vi "ReadMultipleDigitalOutputs.vi"(8 "error in (no error)":errorcluster, 11 "TesteractHAL_DigitalOutput_NIDAQmx In":refnum<class "TesteractHAL_DigitalOutput_NIDAQmx.lvclass">) -> (0 "error out":errorcluster, 2 "data":bool[](array[boolean]), 3 "TesteractHAL_DigitalOutput_NIDAQmx Out":refnum<class "TesteractHAL_DigitalOutput_NIDAQmx.lvclass">)   [LabVIEW 2017, in "TesteractHAL_DigitalOutput_NIDAQmx.lvlib" / "TesteractHAL_DigitalOutput_NIDAQmx.lvclass"]
doc: "Read multiple lines as booleans"
uses:
  TesteractHAL_DigitalOutput_NIDAQmx.lvclass
  TesteractHAL_DigitalOutput_NIDAQmx.lvclass/TesteractHAL_DigitalOutput_NIDAQmx.ctl
  <vilib>/DAQmx/read.llb/DAQmx Read (Digital Bool 1Line 1Point).vi
  <vilib>/DAQmx/create/channels.llb/DAQmx Create Channel (DO-Digital Output).vi
  <vilib>/DAQmx/miscellaneous.llb/DAQmx Fill In Error Info.vi
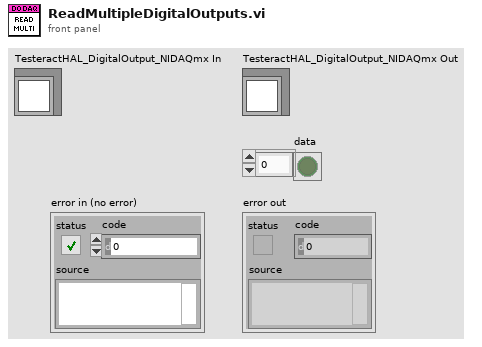
[diagram p1: front panel]
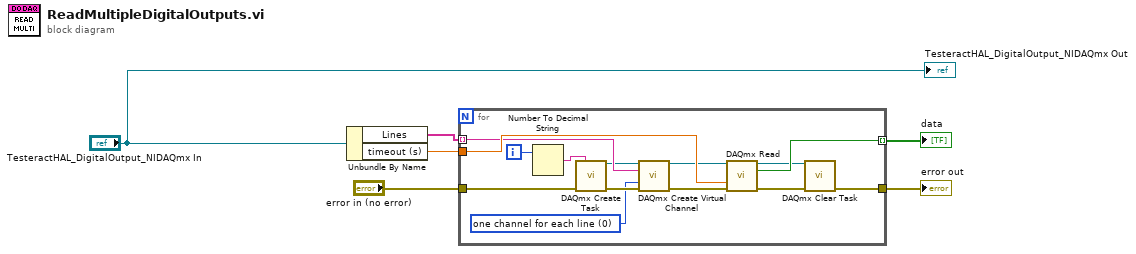
[diagram p0: block diagram]
diagram:
  n1 = Unbundle By Name("TesteractHAL_DigitalOutput_NIDAQmx In") -> ("Lines"=w3:string[], "timeout (s)"=w2:dbl)
  n2 = for {
    tunnel: [w17] -> w6
    tunnel: [w19] -> w5 mode=indexing
    tunnel: w3 -> [w11] mode=indexing
    tunnel: w2 -> [w18]
    tunnel: "error in (no error)" -> [w9]
    i -> [w13]
    w7 = 0 items=["one channel for each line", "one channel for all lines"] ("line grouping")
    n3 = Number To Decimal String(number=w13) -> (decimal integer string=w12:string)  [unwired: 1 in]
    n4 = call <vilib>:"DAQmx Create Task.vi"("new task name"=w12, "error in"=w9) -> ("task out"=w10:refnum<k21>, "error out"=w8:errorcluster)  [unwired: 12 in]
    n5 = call-poly <vilib>:"DAQmx Create Virtual Channel.vi"("task in"=w10, "lines"=w11, "line grouping"=w7, "error in"=w8) -> ("task out"=w14:refnum<k21>, "error out"=w15:errorcluster)  [unwired: 10 in]
    n6 = call-poly <vilib>:"DAQmx Read.vi"("task/channels in"=w14, "timeout"=w18, "error in"=w15) -> ("task out"=w16:refnum<k21>, "data"=w19:bool, "error out"=w20:errorcluster)  [unwired: 10 in]
    n7 = call <vilib>:"DAQmx Clear Task.vi"("task in"=w16, "error in"=w20) -> ("error out"=w17:errorcluster)  [unwired: 13 in]
  }
  "error out" <- w6
  "data" <- w5
  "TesteractHAL_DigitalOutput_NIDAQmx Out" <- "TesteractHAL_DigitalOutput_NIDAQmx In"
